vi "Application Example_Simple.vi"() -> ()   [LabVIEW 2019]
uses:
  Engine/SubVIs/GMLAN/_SubVIs/DTCStatusMask.ctl
  _SubVIs/DPID Parameters.ctl
  _SubVIs/DPID Periodic Rate.ctl
  <vilib>/Automotive Diagnostic Command Set/Diagnostic Protocols.llb/Diagnostic Trouble Code.ctl
  <vilib>/Automotive Diagnostic Command Set/Diagnostic Protocols.llb/DTC Descriptor.ctl
  Engine/SubVIs/GMLAN/_SubVIs/ReadDataByPacketIdentifier_SubFunctions.ctl
  Engine/SubVIs/GMLAN/_SubVIs/DisableNormalCommunication_Parameter.ctl
  Engine/SubVIs/GMLAN/_SubVIs/ReadDiagnosticInformation_ByStatus.vi
  Engine/SubVIs/GMLAN/Utilities/Convert Raw Data to DTCs.vi
  <vilib>/Utility/error.llb/Clear Errors.vi
  Engine/SubVIs/GMLAN/Utilities/GMLAN Service Broadcast.vi
  <vilib>/Automotive Diagnostic Command Set/Diagnostic Transport.llb/Diagnostic Service Send.vi
  <vilib>/Automotive Diagnostic Command Set/Diagnostic Transport.llb/Diagnostic Response Recv.vi
  <vilib>/Automotive Diagnostic Command Set/Diagnostic Transport.llb/ISOTP Transmit.vi
  <vilib>/Automotive Diagnostic Command Set/Diagnostic Transport.llb/ISOTP7 Transmit.vi
  <vilib>/Automotive Diagnostic Command Set/Diagnostic Transport.llb/DoIP Transmit.vi
  <vilib>/Automotive Diagnostic Command Set/Diagnostic Transport.llb/LIN ISOTP Transmit.vi
  <vilib>/Automotive Diagnostic Command Set/Diagnostic Transport.llb/Diagnostic Service Recv.vi
  <vilib>/Automotive Diagnostic Command Set/Diagnostic Transport.llb/ISOTP Send FF.vi
  <vilib>/Automotive Diagnostic Command Set/Diagnostic Transport.llb/ISOTP Send CFs.vi
  <vilib>/Automotive Diagnostic Command Set/Diagnostic Transport.llb/ISOTP Send Frame.vi
  <vilib>/Automotive Diagnostic Command Set/Diagnostic Transport.llb/ISOTP7 Send FF.vi
  <vilib>/Automotive Diagnostic Command Set/Diagnostic Transport.llb/ISOTP7 Send CFs.vi
  <vilib>/Automotive Diagnostic Command Set/Diagnostic Transport.llb/ISOTP7 Send Frame.vi
  <vilib>/Automotive Diagnostic Command Set/Diagnostic Transport.llb/DoIP TCP Msg Send.vi
  <vilib>/Automotive Diagnostic Command Set/Diagnostic Transport.llb/DoIP TCP Msg Recv.vi
  <vilib>/Automotive Diagnostic Command Set/Diagnostic Transport.llb/DoIP Check Addresses.vi
  <vilib>/Automotive Diagnostic Command Set/Diagnostic Transport.llb/DoIP Check ACK Code.vi
  <vilib>/Automotive Diagnostic Command Set/Diagnostic Transport.llb/ISOTP Receive.vi
  <vilib>/Automotive Diagnostic Command Set/Diagnostic Transport.llb/ISOTP7 Receive.vi
  <vilib>/Automotive Diagnostic Command Set/Diagnostic Transport.llb/DoIP Receive.vi
  <vilib>/Automotive Diagnostic Command Set/Diagnostic Transport.llb/LIN ISOTP Receive.vi
  <vilib>/Automotive Diagnostic Command Set/Diagnostic Transport.llb/Diag Get Globals.vi
  <vilib>/Automotive Diagnostic Command Set/Diagnostic Transport.llb/ISOTP Recv FC.vi
  <vilib>/Automotive Diagnostic Command Set/Diagnostic Transport.llb/ISOTP Send CF.vi
  <vilib>/Automotive Diagnostic Command Set/Diagnostic Transport.llb/Diag Fill Frame.vi
  <vilib>/Automotive Diagnostic Command Set/Diagnostic Transport.llb/ISOTP Calc Send Params.vi
  <vilib>/Automotive Diagnostic Command Set/Diagnostic Transport.llb/ISOTP7 Recv FC.vi
  <vilib>/Automotive Diagnostic Command Set/Diagnostic Transport.llb/ISOTP7 Send CF.vi
  <vilib>/Automotive Diagnostic Command Set/Diagnostic Transport.llb/DoIP Add Addresses.vi
  <vilib>/Automotive Diagnostic Command Set/Diagnostic Transport.llb/DoIP TCP Send.vi
  <vilib>/Automotive Diagnostic Command Set/Diagnostic Transport.llb/DoIP TCP Recv.vi
  <vilib>/Automotive Diagnostic Command Set/Diagnostic Transport.llb/DoIP Add Header.vi
  <vilib>/Automotive Diagnostic Command Set/Diagnostic Transport.llb/ISOTP Recv Frame.vi
  <vilib>/Automotive Diagnostic Command Set/Diagnostic Transport.llb/ISOTP Recv CFs.vi
  <vilib>/Automotive Diagnostic Command Set/Diagnostic Transport.llb/ISOTP7 Recv Frame.vi
  <vilib>/Automotive Diagnostic Command Set/Diagnostic Transport.llb/ISOTP7 Recv CFs.vi
  <vilib>/Automotive Diagnostic Command Set/Diagnostic Transport.llb/DoIP Send Alive.vi
  <vilib>/Automotive Diagnostic Command Set/Diagnostic Transport.llb/DoIP Check Error.vi
  <vilib>/Automotive Diagnostic Command Set/Diagnostic Transport.llb/ISOTP Check Redo.vi
  <vilib>/Automotive Diagnostic Command Set/Diagnostic Transport.llb/ISOTP Recv Block.vi
  <vilib>/Automotive Diagnostic Command Set/Diagnostic Transport.llb/ISOTP7 Recv Block.vi
  <vilib>/Automotive Diagnostic Command Set/Diagnostic Transport.llb/ISOTP Send FC.vi
  <vilib>/Automotive Diagnostic Command Set/Diagnostic Transport.llb/ISOTP Add CF.vi
  <vilib>/Automotive Diagnostic Command Set/Diagnostic Transport.llb/ISOTP7 Send FC.vi
  <vilib>/Automotive Diagnostic Command Set/Diagnostic Transport.llb/ISOTP7 Add CF.vi
  <vilib>/Automotive Diagnostic Command Set/Diagnostic Transport.llb/Diagnostic Service.vi
  <vilib>/Automotive Diagnostic Command Set/Diagnostic Transport.llb/Apply Success Failure Error.vi
  <vilib>/Automotive Diagnostic Command Set/Diagnostic Transport.llb/Diag Globals.vi
  <vilib>/Automotive Diagnostic Command Set/Diagnostic Transport.llb/CAN Send Frame Check Queue.vi
  <vilib>/Automotive Diagnostic Command Set/Diagnostic Transport.llb/Diag CAN get timestamp.vi
  <vilib>/Automotive Diagnostic Command Set/Diagnostic Transport.llb/Diag CAN read.vi
  <vilib>/Automotive Diagnostic Command Set/Diagnostic Transport.llb/ISOTP Calc Actual IO Mode.vi
  <vilib>/Automotive Diagnostic Command Set/Diagnostic Transport.llb/ISOTP Get FC Data.vi
  <vilib>/Automotive Diagnostic Command Set/Diagnostic Transport.llb/VWTP Write.vi
  <vilib>/Automotive Diagnostic Command Set/Diagnostic Transport.llb/DoIP Analyze Header.vi
  <vilib>/Automotive Diagnostic Command Set/Diagnostic Transport.llb/Diag CAN status.vi
  <vilib>/Automotive Diagnostic Command Set/Diagnostic Transport.llb/VWTP Read.vi
  <vilib>/Automotive Diagnostic Command Set/Diagnostic Transport.llb/Apply Diagnostic Error.vi
  <vilib>/Automotive Diagnostic Command Set/Diagnostic Protocols.llb/Convert to Phys.vi
  Engine/SubVIs/GMLAN/GMLAN.lvlib
panel:
  in  "DTC Reset":bool
  in  "stop":bool
  in  "Enable Comm 2":bool
  out "Success?":bool=TRUE
  out "stopped?":bool=TRUE
  in  "Read DID":bool
  in  "Read DTCs":bool
  in  "Tab Control":T1(tab)
  in  "CAN Interface":string(combo)="CAN1"
  in  "Baudrate":u32=500000
  in  "Receive ID":u32=2024 format="%.0x"
  in  "Transmit ID":u32=2016 format="%.0x"
  in  "UUDT Receive ID":u32=1512 format="%.0x"
  in  "DPIDs":T3(array[cluster])=[{"DPID ID"=239, "Speed"=enum."Medium", "PIDs"=[14]}, {"DPID ID"=253, "Speed"=enum."Fast", "PIDs"=[12]}] {"PIDs" format="%.0x"; "DPID ID" format="%.0x"}
  in  "DTC descriptor":T4={"DTC Byte Length"=2, "Status Byte Length"=1, "Add Data Byte Length"=1, "Byte Order"=enum."Motorola"}
  in  "DID ID":u8=153 format="%.0x"
  out "DID Data":u8[](array[numeric])=[32, 8, 18, 17]
  out "PID Data":u8[](array[numeric])=[128]
  in  "PID ID":u16=14 format="%.0x"
  in  "CPID ID":u8=29 format="%.0x"
  in  "CPIDControlBytes":u8[](array[numeric])=[0, 0, 0, 0, 0] format="%.0x"
  out "DPID":T5={"DPID ID"=253, "Speed"=enum."Fast", "PIDs"=[12]}
  out "timestamp":timestamp=timestamp(3432175878.295675 s since 1904-01-01)
  out "payload":u8[](array[numeric])
  out "DTCs":T6[](array[typedef])
  in  "status mask":T7={"DTC supported by calibration"=FALSE, "current DTC"=TRUE, "test not passed since DTC cleared"=FALSE, "test failed since DTC cleared"=FALSE, "history DTC"=FALSE, "test not passed since current power up"=FALSE, "current DTC since power up"=FALSE, "warning indicator requested state"=FALSE}
  out "ChangeDTCCount":u16
  out "error IO":errorcluster
  in  "Setup DPIDs":bool
  in  "Stop DPIDs":bool
  in  "Start DPIDs":bool
  in  "Read PIDs":bool
  in  "Write CPID":bool
  in  "Disable Comm":bool
  in  "Enable Comm":bool
  # "$90 - VehicleIdentificationNumber (VIN)\n$92\t- System Supplier ID\n$97\t- SystemNameOrEngineType"
  # "$C - Engine Speed\n$E\t- Spark Advance"
  # "x10 CDAR\nx1D PHSR"
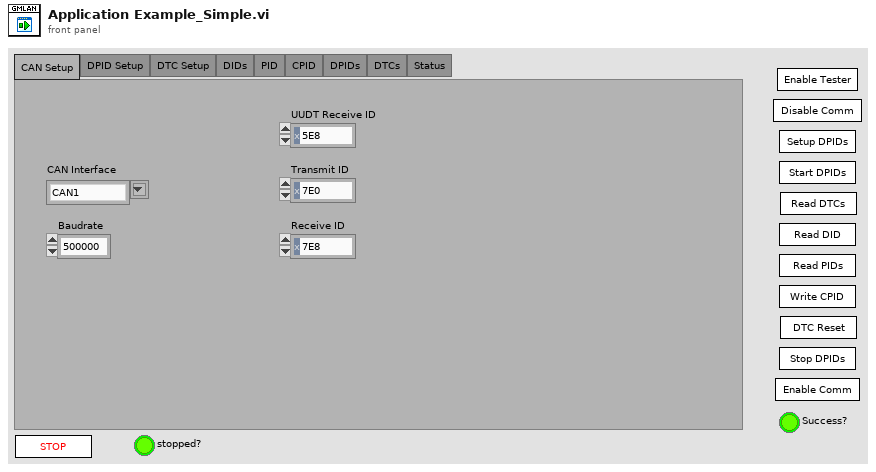
[diagram p1: front panel]
types:
  T1 = enum32{"CAN Setup", "DPID Setup", "DTC Setup", "DIDs", "PID", "CPID", "DPIDs", "DTCs", "Status"}
  T2 = typedef "DPID Periodic Rate.ctl" = enum16{"Slow", "Medium", "Fast"}
  T3 = cluster{"DPID ID":u8, "Speed":T2, "PIDs":u16[]}[]
  T4 = typedef "DTC Descriptor.ctl" = cluster{"DTC Byte Length":i32, "Status Byte Length":i32, "Add Data Byte Length":i32, "Byte Order":enum16{"Motorola", "Intel"}}
  T5 = typedef "DPID Parameters.ctl" = cluster{"DPID ID":u8, "Speed":T2, "PIDs":u16[]}
  T6 = typedef "Diagnostic Trouble Code.ctl" = cluster{"DTC":u32, "Status":u32, "Add Data":u32}
  T7 = typedef "GMLAN.lvlib/DTCStatusMask.ctl" = cluster{"DTC supported by calibration":bool, "current DTC":bool, "test not passed since DTC cleared":bool, "test failed since DTC cleared":bool, "history DTC":bool, "test not passed since current power up":bool, "current DTC since power up":bool, "warning indicator requested state":bool}
  T8 = typedef "GMLAN.lvlib/UUDT Engine Refs.ctl" = cluster{"Engine Ref":refnum<vi>, "UUDT Receive ID":u32}
  T9 = typedef "NI_Automotive Diagnostic Command Set.lvlib/Diag Reference.ctl" = cluster{"Diag CAN Handle":u32, "Transport Protocol":T10, "Receive Address Extension":u8, "Transmit Address Extension":u8, "Receive CAN Id":u32, "Transmit CAN Id":u32, "Log Frames ?":bool, "My TP Address":u8, "Other TP Address":u8, "T1":u16, "T2":u16, "T3":u16, "T4":u16, "Tx SN":u8, "Block Size":u8, "Rx SN":u8, "VW TP Initialized?":bool, "Tx block no":u8, "baud rate":u64, "Interface":string, "Channel Diag CAN Handle":u32, "UDP Connection ID":refnum<k16>, "TCP Connection ID":refnum<k5>, "Target IP Addr":u32, "Source Address":u16, "Target Address":u16, "Send Header NACK?":bool, "DLL Handle":u32, "NAD":u8, "Time Stamp read first":dbl, "Time Stamp read last":dbl, "Time Stamp write first":dbl, "Time Stamp write last":dbl, "Time Stamp write":dbl, "Time Stamp read":dbl, " I/O Mode":u32, "FD Baudrate":u64, "TX_DL":u16, "RX_DL":u16, "DoIP Protocol Version":T11, " Selected I/O Mode":u32, "TesterPresent Counter":u32, "TesterPresent Limit":u32, "TesterPresent Tick[ms]":i32, "TesterPresent RequireResponse?":bool, "TesterPresent Stored Ref?":bool, "TesterPresent Message":u8[], "TesterPresent Task Handle":i32, "TesterPresent Semaphore":T12, "Response Plausibility Check":u32, "Default Version?":bool, "Diagostic Globals":T13, "Session-based Properties?":bool}
  T10 = typedef "NI_Automotive Diagnostic Command Set.lvlib/Transport Protocol Selector.ctl" = enum16{"ISO TP - Normal Mode", "ISO TP - Mixed Mode", "VW TP 2.0", "Diagnostics on IP", "ISO TP LIN"}
  T11 = typedef "NI_Automotive Diagnostic Command Set.lvlib/DoIP Protocol Version.ctl" = u8
  T12 = typedef "Semaphore RefNum" = refnum<k1>
  T13 = typedef "NI_Automotive Diagnostic Command Set.lvlib/Diag Globals.ctl" = cluster{"Timeout FC (Bs)":u32, "Timeout CF (Cr)":u32, "Timeout Diag Command":u32, "Receive Block Size (BS)":u8, "Wait Time CF (STmin)":u8, "Max Waits (N_WFTmax)":u8, "Waits to Send (N_WAIT)":i32, "Time between Waits (TW)":u32, "Fill CAN Frames?":bool, "Fill Byte":u32, "Invalid Response as Error?":bool, "Max RspPending Count":u32, "VWTP Command Timeout":u32, "Transport Protocol":T10, "Diag CAN Handle":u32, "DLL Handle":u32, "Timeout RspPending":u32}
  T14 = enum8{"Idle", "Read DID", "Read DTCs", "Reset DTCs", "Setup DPIDs", "Start DPIDs", "Stop DPIDs", "Read PID", "Write CPID", "DisableCommunication", "EnableCommunication", "Stop"}
  T15 = typedef "GMLAN.lvlib/ReadDataByPacketIdentifier_SubFunctions.ctl" = enum8{"stopSending", "sendOneResponse", "scheduleAtSlowRate", "scheduleAtMediumRate", "scheduleAtFastRate"}
  T16 = typedef "GMLAN.lvlib/DisableNormalCommunication_Parameter.ctl" = enum8{"SpecificECU", "EntireNetwork"}
  T17 = typedef "Filtered DPID IDs.ctl" = cluster{"Slow":u8[], "Medium":u8[], "Fast":u8[]}
  T18 = typedef "GMLAN.lvlib/UUDT Messages.ctl" = cluster{"UUDT Reponses":T19, "Data":T20[]}
  T19 = typedef "GMLAN.lvlib/UUDT Responses.ctl" = enum16{"DPID", "DTCStatus", "DTCReport", "ChangeDTCCount"}
  T20 = typedef "XNET Frame CAN.ctl" = cluster{"timestamp":timestamp, "payload":u8[], "identifier":u32, "type":T21, "extended?":bool, "echo?":bool}
  T21 = typedef "XNET Frame Type CAN.ctl" = u8
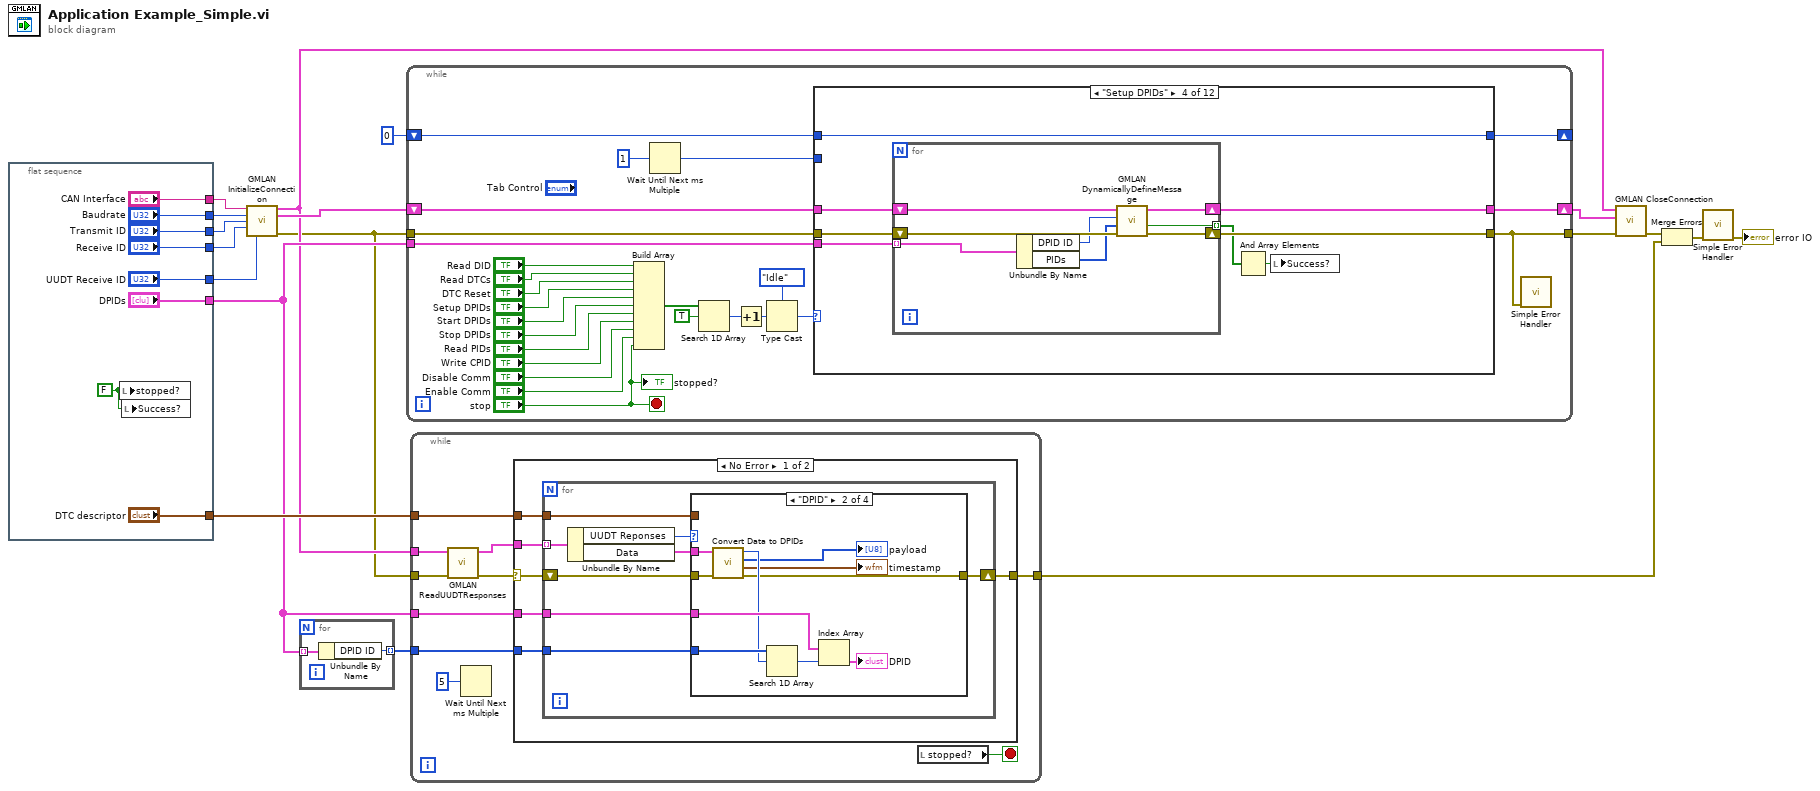
[diagram p0: block diagram]
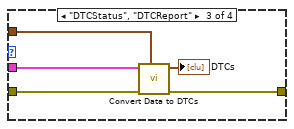
[diagram p3: hidden frame]
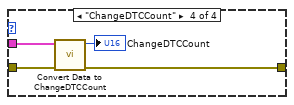
[diagram p4: hidden frame]
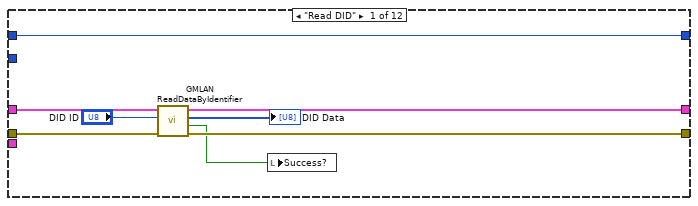
[diagram p6: hidden frame]
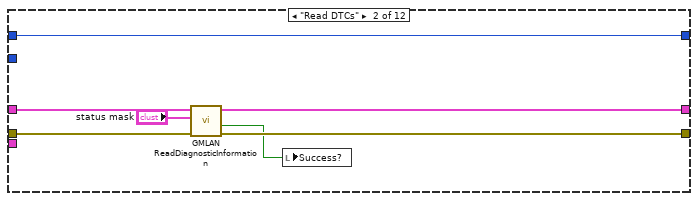
[diagram p7: hidden frame]
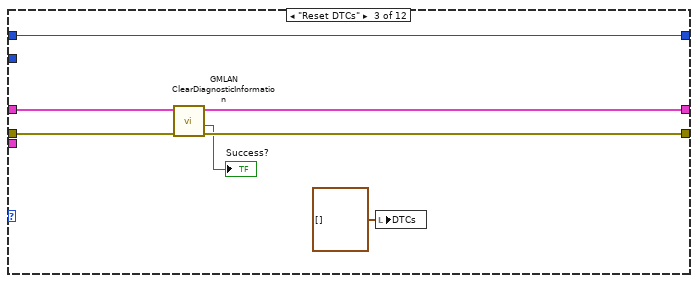
[diagram p8: hidden frame]
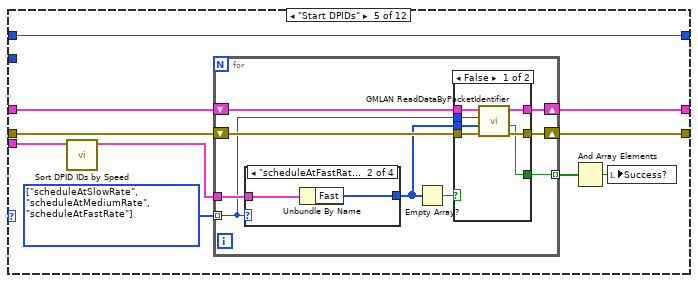
[diagram p9: hidden frame]
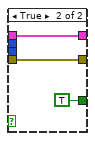
[diagram p10: hidden frame]
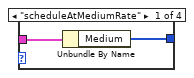
[diagram p11: hidden frame]
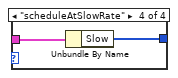
[diagram p13: hidden frame]
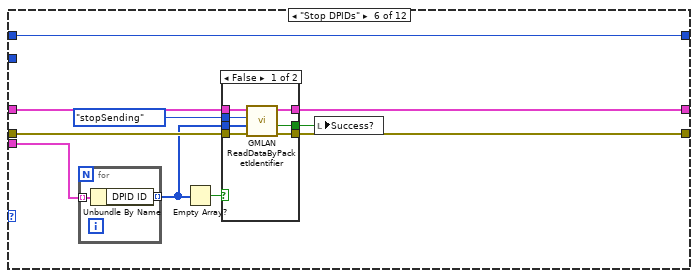
[diagram p14: hidden frame]
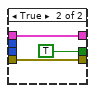
[diagram p15: hidden frame]
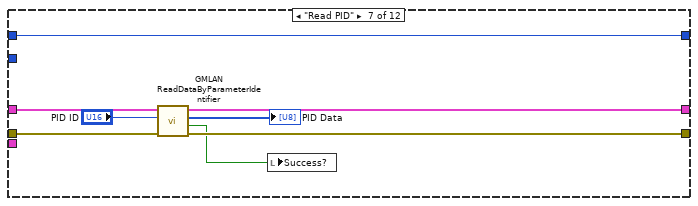
[diagram p16: hidden frame]
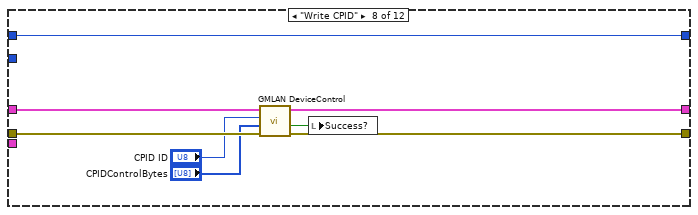
[diagram p17: hidden frame]
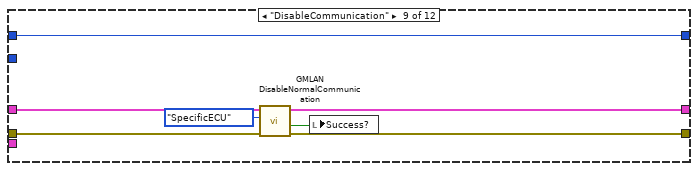
[diagram p18: hidden frame]
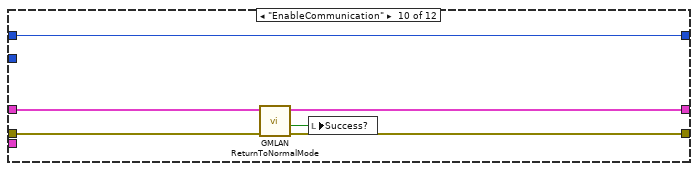
[diagram p19: hidden frame]
diagram:
  n1 = flat-sequence {
    tunnel: ["Baudrate"] -> w8
    tunnel: ["Transmit ID"] -> w5
    tunnel: ["Receive ID"] -> w7
    tunnel: ["UUDT Receive ID"] -> w6
    tunnel: ["DTC descriptor"] -> w18
    tunnel: ["DPIDs"] -> w17
    tunnel: ["CAN Interface"] -> w9
    frame #0 {
      w20 = FALSE ("stopped?")
      n2 = local write "stopped?"(w20) -> ()
      n3 = local write "Success?"(w20) -> ()
    }
  }
  n4 = call "GMLAN InitializeConnection.vi"("CAN Interface"=w9, "Baudrate"=w8, "Transmit ID"=w5, "Receive ID"=w7, "UUDT Receive ID"=w6) -> ("UUDT Engine"=w2:T8, "ADCS Ref"=w3:T9, "error out"=w1:errorcluster)  [unwired: 8 in]
  n5 = for {
    tunnel: w17 -> [w28] mode=indexing
    tunnel: [w27] -> w11 mode=indexing
    n6 = Unbundle By Name(w28) -> ("DPID ID"=w27:u8)
  }
  n7 = while {
    tunnel: w1 -> [w53]
    tunnel: [w32] -> w10
    shift-right: [w52] -> w4
    shift-left: w3 -> [w54]
    shift-right: [w46] -> _
    shift-left: u32 0 ("millisecond timer value") -> [w44]
    tunnel: w17 -> [w40]
    stop <- "stop" stop-if-true
    n8 = Build Array("Read DID", "Read DTCs", "DTC Reset", "Setup DPIDs", "Start DPIDs", "Stop DPIDs", "Read PIDs", "Write CPID", "Disable Comm", "Enable Comm", "stop") -> (w50:bool[])
    n9 = Wait Until Next ms Multiple(millisecond multiple=1) -> (millisecond timer value=w45:u32)
    n10 = Search 1D Array(1D array=w50, element=TRUE) -> (index of element=w37:i32)  [unwired: 1 in]
    n11 = Increment(x=w37) -> (x+1=w35:u8)
    n12 = Type Cast(type=T14."Idle", x=w35) -> (*(type *) &x=w34:T14)
    n13 = case shown="\"Setup DPIDs\"" w34 {
      tunnel: w54 -> [w62 w68 w76 w81 w100 w135 w157 w164 w171 w177 w179 w192]
      tunnel: w53 -> [w61 w66 w75 w83 w102 w137 w156 w165 w172 w178 w180 w193]
      tunnel: [w60 w64 w74 w80 w99 w134 w155 w162 w169 w175 w179 w190] -> w52
      tunnel: [w59 w65 w73 w82 w101 w136 w154 w163 w170 w176 w180 w191] -> w32
      tunnel: w45 -> [_ _ _ _ _ _ _ _ _ _ _ w188]
      tunnel: [w55 w69 w72 w84 w98 w133 w150 w161 w168 w174 w181 w189] -> w46
      tunnel: w44 -> [w55 w69 w72 w84 w98 w133 w150 w161 w168 w174 w181 w184]
      tunnel: w40 -> [_ _ _ w79 w97 w132 _ _ _ _ _ _]
      frame "Read DID" {
        n14 = call "GMLAN ReadDataByIdentifier.vi"("error in (no error)"=w61, "Data ID (DID)"="DID ID", "diag ref in"=w62) -> ("error out"=w59:errorcluster, "success?"=w58:bool, "data out"=→"DID Data":u8[], "diag ref out"=w60:T9)  [unwired: 5 in]
        n15 = local write "Success?"(w58) -> ()
      }
      frame "Read DTCs" {
        n16 = call-poly "GMLAN ReadDiagnosticInformation.vi"("error in (no error)"=w66, "status mask"="status mask", "diag ref in"=w68) -> ("error out"=w65:errorcluster, "success?"=w63:bool, "diag ref out"=w64:T9)  [unwired: 5 in, 1 out]
        n17 = local write "Success?"(w63) -> ()
      }
      frame "Reset DTCs" {
        n18 = call "GMLAN ClearDiagnosticInformation.vi"("error in (no error)"=w75, "diag ref in"=w76) -> ("error out"=w73:errorcluster, "success?"=→"Success?":bool, "diag ref out"=w74:T9)  [unwired: 7 in]
        n19 = local write "DTCs"(T6[] [] ("DTCs")) -> ()
      }
      frame "Setup DPIDs" {
        n20 = for {
          shift-right: [w91] -> w82
          shift-left: w83 -> [w92]
          shift-right: [w89] -> w80
          shift-left: w81 -> [w90]
          tunnel: w79 -> [w88] mode=indexing
          tunnel: [w85] -> w78 mode=indexing
          n21 = Unbundle By Name(w88) -> ("DPID ID"=w87:u8, "PIDs"=w86:u16[])
          n22 = call "GMLAN DynamicallyDefineMessage.vi"("error in (no error)"=w92, "PID List"=w86, "DPID ID"=w87, "diag ref in"=w90) -> ("error out"=w91:errorcluster, "success?"=w85:bool, "diag ref out"=w89:T9)  [unwired: 5 in]
        }
        n23 = And Array Elements(Boolean array=w78) -> (logical AND=w77:bool)
        n24 = local write "Success?"(w77) -> ()
      }
      frame "Start DPIDs" {
        w95 = T15[] [enum."scheduleAtSlowRate", enum."scheduleAtMediumRate", enum."scheduleAtFastRate"] items=["stopSending", "sendOneResponse", "scheduleAtSlowRate", "scheduleAtMediumRate", "scheduleAtFastRate"]
        n25 = call "Sort DPID IDs by Speed.vi"("DPIDs"=w97) -> ("Filtered DPIDs IDs"=w96:T17)  [unwired: 10 in]
        n26 = for {
          tunnel: w96 -> [w107]
          shift-right: [w110] -> w101
          shift-left: w102 -> [w111]
          shift-right: [w108] -> w99
          shift-left: w100 -> [w109]
          tunnel: w95 -> [w104] mode=indexing
          tunnel: [w103] -> w93 mode=indexing
          n27 = case shown="\"scheduleAtFastRate\"" w104 {
            tunnel: w107 -> [w123 w125 _ w127]
            tunnel: [w122 w124 _ w126] -> w106
            frame "scheduleAtMediumRate" {
              n28 = Unbundle By Name(w123) -> ("Medium"=w122:u8[])
            }
            frame "scheduleAtFastRate" {
              n29 = Unbundle By Name(w125) -> ("Fast"=w124:u8[])
            }
            frame Default {
            }
            frame "scheduleAtSlowRate" {
              n30 = Unbundle By Name(w127) -> ("Slow"=w126:u8[])
            }
          }
          n31 = Empty Array?(array=w106) -> (empty?=w105:bool)
          n32 = case shown="False" w105 {
            tunnel: w111 -> [w118 w120]
            tunnel: [w117 w120] -> w110
            tunnel: w109 -> [w116 w121]
            tunnel: [w115 w121] -> w108
            tunnel: w104 -> [w114 _]
            tunnel: w106 -> [w113 _]
            tunnel: [w112 TRUE ("success?")] -> w103
            frame False {
              n33 = call "GMLAN ReadDataByPacketIdentifier.vi"("error in (no error)"=w118, "DPIDs"=w113, "Sub Function"=w114, "diag ref in"=w116) -> ("error out"=w117:errorcluster, "success?"=w112:bool, "diag ref out"=w115:T9)  [unwired: 4 in, 1 out]
            }
            frame True {
            }
          }
        }
        n34 = And Array Elements(Boolean array=w93) -> (logical AND=w94:bool)
        n35 = local write "Success?"(w94) -> ()
      }
      frame "Stop DPIDs" {
        n36 = for {
          tunnel: w132 -> [w149] mode=indexing
          tunnel: [w148] -> w130 mode=indexing
          n37 = Unbundle By Name(w149) -> ("DPID ID"=w148:u8)
        }
        n38 = Empty Array?(array=w130) -> (empty?=w131:bool)
        n39 = case shown="False" w131 {
          tunnel: w137 -> [w144 w146]
          tunnel: [w143 w146] -> w136
          tunnel: w135 -> [w142 w147]
          tunnel: [w141 w147] -> w134
          tunnel: ReadDataByPacketIdentifier_SubFunctions."stopSending" ("Sub Function") -> [w140 _]
          tunnel: w130 -> [w139 _]
          tunnel: [w138 TRUE ("success?")] -> w128
          frame False {
            n40 = call "GMLAN ReadDataByPacketIdentifier.vi"("error in (no error)"=w144, "DPIDs"=w139, "Sub Function"=w140, "diag ref in"=w142) -> ("error out"=w143:errorcluster, "success?"=w138:bool, "diag ref out"=w141:T9)  [unwired: 4 in, 1 out]
          }
          frame True {
          }
        }
        n41 = local write "Success?"(w128) -> ()
      }
      frame "Read PID" {
        n42 = call "GMLAN ReadDataByParameterIdentifier.vi"("error in (no error)"=w156, "Parameter ID (PID)"="PID ID", "diag ref in"=w157) -> ("error out"=w154:errorcluster, "success?"=w153:bool, "data out"=→"PID Data":u8[], "diag ref out"=w155:T9)  [unwired: 5 in]
        n43 = local write "Success?"(w153) -> ()
      }
      frame "Write CPID" {
        n44 = call "GMLAN DeviceControl.vi"("error in (no error)"=w165, "CPIDControlBytes"="CPIDControlBytes", "CPID ID"="CPID ID", "diag ref in"=w164) -> ("error out"=w163:errorcluster, "success?"=w160:bool, "diag ref out"=w162:T9)  [unwired: 5 in]
        n45 = local write "Success?"(w160) -> ()
      }
      frame "DisableCommunication" {
        n46 = call "GMLAN DisableNormalCommunication.vi"("error in (no error)"=w172, "Parameter"=DisableNormalCommunication_Parameter."SpecificECU", "diag ref in"=w171) -> ("error out"=w170:errorcluster, "success?"=w166:bool, "diag ref out"=w169:T9)  [unwired: 6 in]
        n47 = local write "Success?"(w166) -> ()
      }
      frame "EnableCommunication" {
        n48 = call "GMLAN ReturnToNormalMode.vi"("error in (no error)"=w178, "diag ref in"=w177) -> ("error out"=w176:errorcluster, "success?"=w173:bool, "diag ref out"=w175:T9)  [unwired: 7 in]
        n49 = local write "Success?"(w173) -> ()
      }
      frame "Stop" {
      }
      frame Default {
        # "Tester Present"
        n50 = Subtract(x=w188, y=w184) -> (x-y=w187:u32)
        n51 = Greater Or Equal?(x=w187, y=u32 1000) -> (x >= y?=w185:bool)
        n52 = Compound Arithmetic op=AND(w185, "Enable Comm 2") -> (w183:bool)
        n53 = case shown="True" w183 {
          tunnel: w193 -> [w195 w201]
          tunnel: w192 -> [w196 w200]
          tunnel: [w195 w199] -> w191
          tunnel: [w196 w198] -> w190
          tunnel: w188 -> [_ w197]
          tunnel: [w194 w197] -> w189
          tunnel: w184 -> [w194 _]
          frame False {
          }
          frame True {
            n54 = call "GMLAN TesterPresent.vi"("error in (no error)"=w201, "diag ref in"=w200) -> ("error out"=w199:errorcluster, "diag ref out"=w198:T9)  [unwired: 7 in, 1 out]
          }
        }
      }
    }
    n55 = call <vilib>:"Simple Error Handler.vi"("error in (no error)"=w32) -> ()  [unwired: 4 in, 5 out]
    "stopped?" <- "stop"
  }
  n56 = while {
    tunnel: w1 -> [w205]
    tunnel: w18 -> [w209]
    tunnel: [w208] -> w13
    tunnel: w17 -> [w207]
    tunnel: w11 -> [w206]
    tunnel: w2 -> [w203]
    stop <- w211 stop-if-true
    n57 = call "GMLAN ReadUUDTResponses.vi"("error in"=w205, "UUDT Engine"=w203) -> ("error out"=w204:errorcluster, "Data"=w202:T18[])  [unwired: 8 in]
    n58 = Wait Until Next ms Multiple(millisecond multiple=5) -> ()  [unwired: 1 out]
    n59 = case shown="No Error" w204 {
      selector: w204 -> [w217 w246]
      tunnel: [w216 w246] -> w208
      tunnel: w209 -> [w215 _]
      tunnel: w207 -> [w214 _]
      tunnel: w206 -> [w213 _]
      tunnel: w202 -> [w212 _]
      frame No Error {
        n60 = for {
          shift-right: [w225] -> w216
          shift-left: w217 -> [w220]
          tunnel: w215 -> [w224]
          tunnel: w214 -> [w223]
          tunnel: w213 -> [w222]
          tunnel: w212 -> [w221] mode=indexing
          n61 = Unbundle By Name(w221) -> ("UUDT Reponses"=w219:T19, "Data"=w218:T20[])
          n62 = case shown="\"DPID\"" w219 {
            tunnel: [w226 w227 w237 w242] -> w225
            tunnel: w220 -> [w226 w228 w238 w243]
            tunnel: w224 -> [_ _ w241 _]
            tunnel: w223 -> [_ w234 _ _]
            tunnel: w222 -> [_ w236 _ _]
            tunnel: w218 -> [_ w232 w239 w245]
            frame Default {
            }
            frame "DPID" {
              n63 = call "Convert Data to DPIDs.vi"("error in (no error)"=w228, "Data"=w232) -> ("error out"=w227:errorcluster, "timestamp"=→"timestamp":timestamp, "DPID Payload"=→"payload":u8[], "DPID ID"=w231:u8)  [unwired: 6 in]
              n64 = Search 1D Array(1D array=w236, element=w231) -> (index of element=w235:i32)  [unwired: 1 in]
              n65 = Index Array(array=w234, index=w235) -> (element=→"DPID":cluster{"DPID ID":u8, "Speed":T2, "PIDs":u16[]})
            }
            frame "DTCStatus", "DTCReport" {
              n66 = call "Convert Data to DTCs.vi"("DTC descriptor"=w241, "error in (no error)"=w238, "All DTCs"=w239) -> ("error out"=w237:errorcluster, "DTCs"=→"DTCs":T6[])  [unwired: 7 in]
            }
            frame "ChangeDTCCount" {
              n67 = call "Convert Data to ChangeDTCCount.vi"("error in (no error)"=w243, "Data"=w245) -> ("error out"=w242:errorcluster, "ChangeDTCCount"=→"ChangeDTCCount":u16)  [unwired: 8 in]
            }
          }
        }
      }
      frame Error {
      }
    }
    n68 = local read "stopped?"() -> (w211:bool)
  }
  n69 = call "GMLAN CloseConnection.vi"("error in (no error)"=w10, "diag ref out"=w4, "UUDT Engine"=w2) -> ("error out"=w12:errorcluster)  [unwired: 8 in]
  n70 = Merge Errors(w12, w13) -> (w14:errorcluster)
  n71 = call <vilib>:"Simple Error Handler.vi"("error in (no error)"=w14) -> ("error out"=→"error IO":errorcluster)  [unwired: 1 in, 7 out]
